vi "waaca_runner.vi"(9 "Numeric":dbl) -> (3 "Numeric 2":dbl)   [LabVIEW 2016]
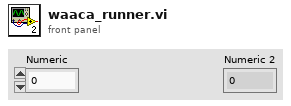
[diagram p1: front panel]
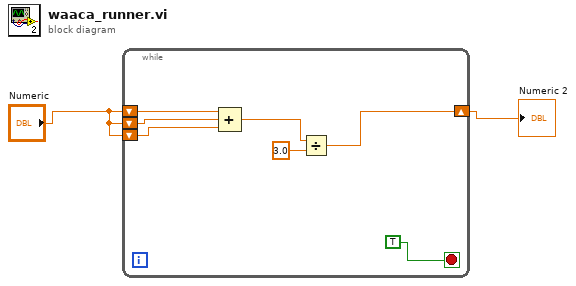
[diagram p0: block diagram]
diagram:
  n1 = while {
    shift-right: [w3] -> w1
    shift-left: "Numeric" -> [w8]
    shift-left: "Numeric" -> [w7]
    shift-left: "Numeric" -> [w6]
    stop <- TRUE stop-if-true
    n2 = Compound Arithmetic op=ADD(w8, w7, w6) -> (w5:dbl)
    n3 = Divide(x=w5, y=3.0) -> (x/y=w3:dbl)
  }
  "Numeric 2" <- w1
